vi "niRFUtil TRC Waveform to Trace (complex WDT).vi"(7 "Complex WDT":T1) -> (8 "Measurement Trace":T2 format="%.2f")   [LabVIEW 2015, in "niRFUtil.lvlib"]
doc: "(c) Copyright 2006, National Instruments, Inc. This VI may not be duplicated, sold, or distributed without written consent from National Instruments."
uses:
  niRFUtil.lvlib
  Includes/niRFUtil INC Trace.ctl
  Includes/niRFUtil INC Complex WDT.ctl
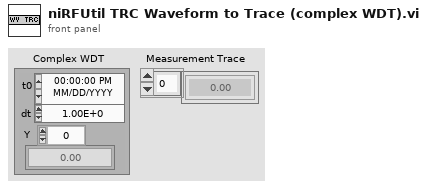
[diagram p1: front panel]
types:
  T1 = typedef "niRFUtil.lvlib/niRFUtil INC Complex WDT.ctl" = waveform(csg)
  T2 = typedef "niRFUtil.lvlib/niRFUtil INC Trace.ctl" = sgl[]
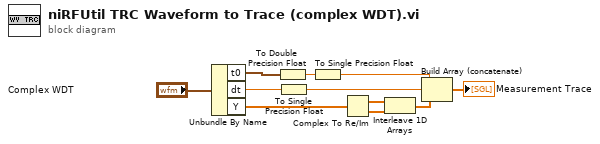
[diagram p0: block diagram]
diagram:
  n1 = Unbundle By Name("Complex WDT") -> ("t0"=w6:timestamp, "dt"=w4:dbl, "Y"=w3:csg[])
  n2 = To Double Precision Float(number=w6) -> (double precision float=w5:dbl)
  n3 = To Single Precision Float(number=w4) -> (single precision float=w1:sgl)
  n4 = To Single Precision Float(number=w5) -> (single precision float=w2:sgl)
  n5 = Complex To Re/Im(x + iy=w3) -> (x=w10:sgl[], y=w11:sgl[])
  n6 = Interleave 1D Arrays(w10, w11) -> (w9:sgl[])
  n7 = Build Array (concatenate)(w2, w1, w9) -> (→"Measurement Trace":sgl[])
